vi "TestiLabview2LowLevel.vi"() -> ()   [LabVIEW 2018]
uses:
  <vilib>/vision/Image Controls.llb/IMAQ Image.ctl
  <vilib>/vision/driver/Vision Acquisition Express Utility VIs.llb/Vision Acquisition Path Convert (Path).vi
  <vilib>/vision/NI_Vision_Development_Module.lvlib
panel:
  out "Isbjerg spottet":i32[](array[numeric])
  out "Y":dbl[][](array[numeric])
  out "X":dbl[][](array[numeric])
  out "Image":T1(plugin-control)
  out "Array":cluster{"X Centroid":sgl, "Y Centroid":sgl}[](array[cluster])
  # "Tager isbjerge i rækkefølgen: y: 0 -> 480"
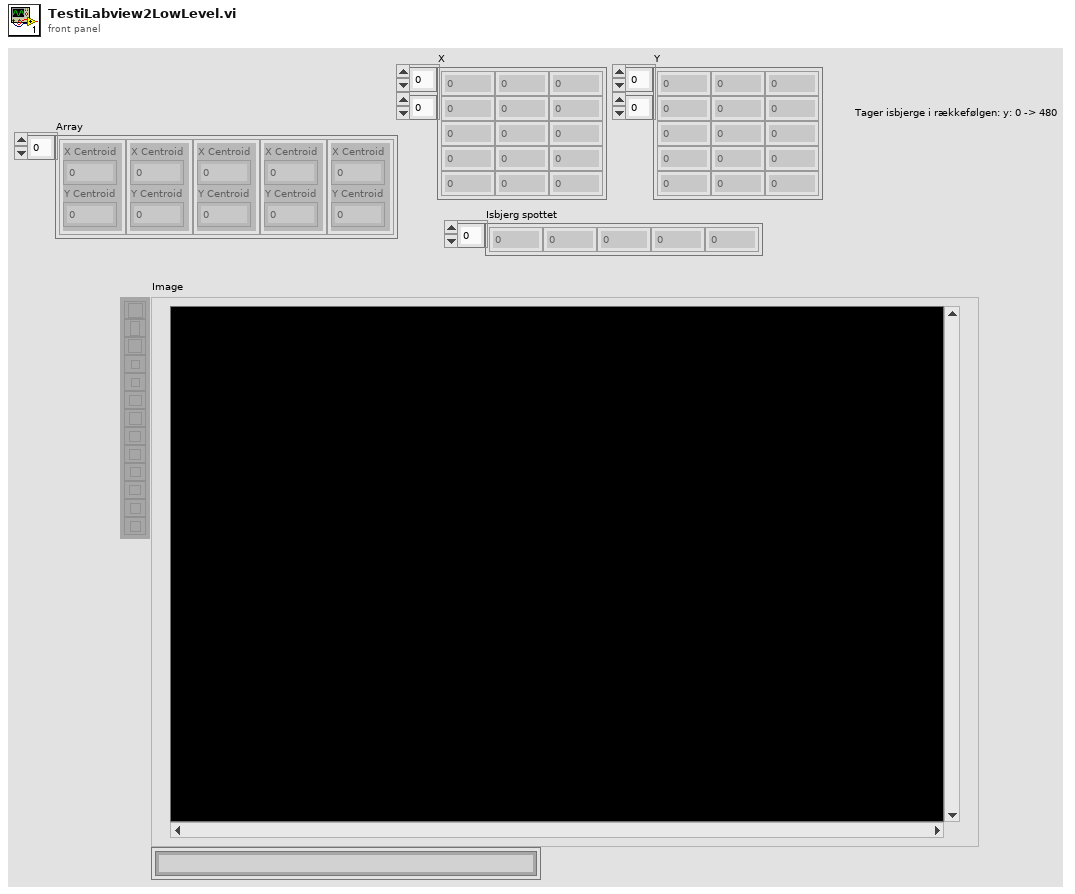
[diagram p1: front panel]
types:
  T1 = typedef "IMAQ Image.ctl" = refnum<image>
  T2 = typedef "Image Type" = u32
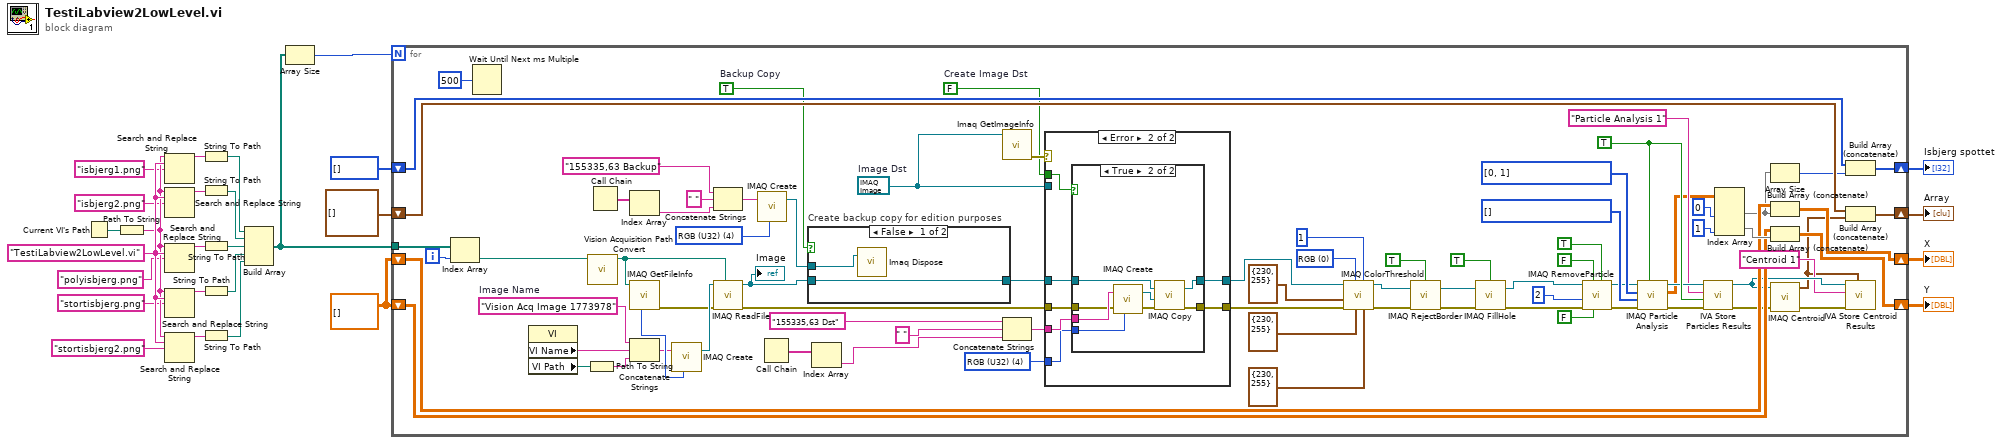
[diagram p0: block diagram]
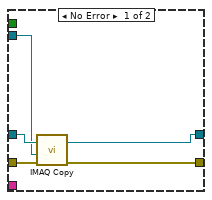
[diagram p2: hidden frame]
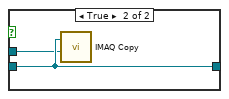
[diagram p4: hidden frame]
diagram:
  w10 = "TestiLabview2LowLevel.vi" ("search string")
  w25 = dbl[][] []
  n1 = Current VI's Path() -> (path=w19:path)
  n2 = Path To String(path=w19) -> (string=w9:string)
  n3 = Search and Replace String(input string=w9, search string=w10, replace string="isbjerg1.png" ("search string")) -> (result string=w18:string)  [unwired: 5 in, 3 out]
  n4 = Search and Replace String(input string=w9, search string=w10, replace string="isbjerg2.png" ("search string")) -> (result string=w17:string)  [unwired: 5 in, 3 out]
  n5 = Search and Replace String(input string=w9, search string=w10, replace string="polyisbjerg.png" ("search string")) -> (result string=w16:string)  [unwired: 5 in, 3 out]
  n6 = Search and Replace String(input string=w9, search string=w10, replace string="stortisbjerg.png" ("search string")) -> (result string=w15:string)  [unwired: 5 in, 3 out]
  n7 = Search and Replace String(input string=w9, search string=w10, replace string="stortisbjerg2.png" ("search string")) -> (result string=w14:string)  [unwired: 5 in, 3 out]
  n8 = String To Path(string=w18) -> (path=w11:path)
  n9 = String To Path(string=w17) -> (path=w12:path)
  n10 = String To Path(string=w16) -> (path=w2:path)
  n11 = String To Path(string=w15) -> (path=w13:path)
  n12 = String To Path(string=w14) -> (path=w1:path)
  n13 = Build Array(w11, w12, w2, w13, w1) -> (w3:path[])
  n14 = Array Size(array=w3) -> (size(s)=w21:i32)
  n15 = for {
    N: w21 -> [_]
    shift-right: [w106] -> w27
    shift-left: cluster{"X Centroid":sgl, "Y Centroid":sgl}[] [] -> [w105]
    tunnel: w3 -> [w103]
    shift-right: [w98] -> w24
    shift-left: w25 -> [w96]
    shift-right: [w97] -> w23
    shift-left: w25 -> [w95]
    shift-right: [w92] -> w20
    shift-left: i32[] [] -> [w91]
    i -> [w104]
    w79 = T1 refnum  # Image Dst
    w41 = i32[] [] items=["Center of Mass X", "Center of Mass Y", "First Pixel X", "First Pixel Y", "Bounding Rect Left", "Bounding Rect Top", "Bounding Rect Right", "Bounding Rect Bottom", "Max Feret Diameter Start X", "Max Feret Diameter Start Y", "Max Feret Diameter End X", "Max Feret Diameter End Y", "Max Horiz. Segment Length Left", "Max Horiz. Segment Length Right", "Max Horiz. Segment Length Row", "-", "Bounding Rect Width", "Bounding Rect Height", "Bounding Rect Diagonal", "Perimeter", "Convex Hull Perimeter", "Holes' Perimeter", "Max Feret Diameter", "Equivalent Ellipse Major Axis", "Equivalent Ellipse Minor Axis", "Equivalent Ellipse Minor Axis (Feret)", "Equivalent Rect Long Side", "Equivalent Rect Short Side", "Equivalent Rect Diagonal", "Equivalent Rect Short Side (Feret)", "Average Horiz. Segment Length", "Average Vert. Segment Length", "Hydraulic Radius", "Waddel Disk Diameter", "-", "Area", "Holes' Area", "Particle & Holes' Area", "Convex Hull Area", "Image Area", "-", "Number of Holes", "Number of Horiz. Segments", "Number of Vert. Segments", "-", "Orientation", "Max Feret Diameter Orientation", "-", "% Area/Image Area", "% Area/(Particle & Holes' Area)", "Ratio of Equivalent Ellipse Axes", "Ratio of Equivalent Rect Sides", "-", "Elongation Factor", "Compactness Factor", "Heywood Circularity Factor", "Type Factor", "-", "Sum X", "Sum Y", "Sum XX", "Sum XY", "Sum YY", "Sum XXX", "Sum XXY", "Sum XYY", "Sum YYY", "-", "Moment of Inertia XX", "Moment of Inertia XY", "Moment of Inertia YY", "Moment of Inertia XXX", "Moment of Inertia XXY", "Moment of Inertia XYY", "Moment of Inertia YYY", "Norm. Moment of Inertia XX", "Norm. Moment of Inertia XY", "Norm. Moment of Inertia YY", "Norm. Moment of Inertia XXX", "Norm. Moment of Inertia XXY", "Norm. Moment of Inertia XYY", "Norm. Moment of Inertia YYY", "Hu Moment 1", "Hu Moment 2", "Hu Moment 3", "Hu Moment 4", "Hu Moment 5", "Hu Moment 6", "Hu Moment 7"] ("Real-World Measurements")
    w42 = i32[] [0, 1] items=["Center of Mass X", "Center of Mass Y", "First Pixel X", "First Pixel Y", "Bounding Rect Left", "Bounding Rect Top", "Bounding Rect Right", "Bounding Rect Bottom", "Max Feret Diameter Start X", "Max Feret Diameter Start Y", "Max Feret Diameter End X", "Max Feret Diameter End Y", "Max Horiz. Segment Length Left", "Max Horiz. Segment Length Right", "Max Horiz. Segment Length Row", "-", "Bounding Rect Width", "Bounding Rect Height", "Bounding Rect Diagonal", "Perimeter", "Convex Hull Perimeter", "Holes' Perimeter", "Max Feret Diameter", "Equivalent Ellipse Major Axis", "Equivalent Ellipse Minor Axis", "Equivalent Ellipse Minor Axis (Feret)", "Equivalent Rect Long Side", "Equivalent Rect Short Side", "Equivalent Rect Diagonal", "Equivalent Rect Short Side (Feret)", "Average Horiz. Segment Length", "Average Vert. Segment Length", "Hydraulic Radius", "Waddel Disk Diameter", "-", "Area", "Holes' Area", "Particle & Holes' Area", "Convex Hull Area", "Image Area", "-", "Number of Holes", "Number of Horiz. Segments", "Number of Vert. Segments", "-", "Orientation", "Max Feret Diameter Orientation", "-", "% Area/Image Area", "% Area/(Particle & Holes' Area)", "Ratio of Equivalent Ellipse Axes", "Ratio of Equivalent Rect Sides", "-", "Elongation Factor", "Compactness Factor", "Heywood Circularity Factor", "Type Factor", "-", "Sum X", "Sum Y", "Sum XX", "Sum XY", "Sum YY", "Sum XXX", "Sum XXY", "Sum XYY", "Sum YYY", "-", "Moment of Inertia XX", "Moment of Inertia XY", "Moment of Inertia YY", "Moment of Inertia XXX", "Moment of Inertia XXY", "Moment of Inertia XYY", "Moment of Inertia YYY", "Norm. Moment of Inertia XX", "Norm. Moment of Inertia XY", "Norm. Moment of Inertia YY", "Norm. Moment of Inertia XXX", "Norm. Moment of Inertia XXY", "Norm. Moment of Inertia XYY", "Norm. Moment of Inertia YYY", "Hu Moment 1", "Hu Moment 2", "Hu Moment 3", "Hu Moment 4", "Hu Moment 5", "Hu Moment 6", "Hu Moment 7"] ("Pixel Measurements")
    w39 = TRUE ("Connectivity 4/8 (8)")
    w60 = u16 0 items=["RGB", "HSL", "HSV", "HSI"] ("Color Mode")
    w62 = T2 4 items=["Grayscale (U8)", "Grayscale (I16)", "Grayscale (SGL)", "Complex (CSG)", "RGB (U32)", "HSL (U32)", "RGB (U64)", "Grayscale (U16)"] ("Image Dst Type")
    w63 = T2 4 items=["Grayscale (U8)", "Grayscale (I16)", "Grayscale (SGL)", "Complex (CSG)", "RGB (U32)", "HSL (U32)", "RGB (U64)", "Grayscale (U16)"] ("Image Type")
    w80 = TRUE  # Backup Copy
    w75 = FALSE  # Create Image Dst
    w84 = "Vision Acq Image 1773978"  # Image Name
    n16 = Index Array(array=w103, index=w104) -> (element=w81:path)
    n17 = Wait Until Next ms Multiple(millisecond multiple=u32 500) -> ()  [unwired: 1 out]
    n18 = property class="VI"() -> ("VI Name"=w86:string, "VI Path"=w87:path)  [unwired: 2 in, 2 out]
    n19 = Path To String(path=w87) -> (string=w85:string)
    n20 = call-poly <vilib>:"Vision Acquisition Path Convert.vi"("Path In"=w81) -> ("Path Out"=w82:path)  [unwired: 10 in]
    n21 = Call Chain() -> (call chain=w69:string[])
    n22 = Index Array(array=w69) -> (element=w68:string)  [unwired: 1 in]
    n23 = call "IMAQ GetFileInfo"("File Path"=w82) -> ("error out"=w88:errorcluster, "Image Type"=w89:T2)  [unwired: 1 in, 8 out]
    n24 = Concatenate Strings(w84, w86, w85) -> (w83:string)
    n25 = call "IMAQ Create"("Image Name"=w83, "Image Type"=w89) -> ("New Image"=w90:T1)  [unwired: 2 in, 2 out]
    n26 = Concatenate Strings("155335,63 Backup" ("Backup Image Name"), " ", w68) -> (w65:string)
    n27 = call "IMAQ ReadFile"("File Path"=w82, "error in (no error)"=w88, "Image"=w90) -> ("error out"=w30:errorcluster, "Image Out"=w31:T1)  [unwired: 2 in, 5 out]
    "Image" <- w31
    n28 = call "IMAQ Create"("Image Name"=w65, "Image Type"=w63) -> ("New Image"=w64:T1)  [unwired: 2 in, 2 out]
    n29 = Call Chain() -> (call chain=w74:string[])
    n30 = case "Create backup copy for edition purposes" shown="False" w80 {
      tunnel: [w130 w132] -> w77
      tunnel: w31 -> [w130 w132]
      tunnel: w64 -> [w129 w131]
      frame False {
        n31 = call "Imaq Dispose"("Image"=w129) -> ()  [unwired: 2 in, 4 out]
      }
      frame True {
        n32 = call "IMAQ Copy"("Image Dst"=w131, "Image Src"=w132) -> ()  [unwired: 1 in, 5 out]
      }
    }
    n33 = Index Array(array=w74) -> (element=w72:string)  [unwired: 1 in]
    n34 = call "Imaq GetImageInfo"("Image"=w79) -> ("error out"=w78:errorcluster)  [unwired: 1 in, 9 out]
    n35 = Concatenate Strings("155335,63 Dst" ("Image Dst Name"), " ", w72) -> (w70:string)
    n36 = case shown="Error" w78 {
      tunnel: [w111 w115] -> w56
      tunnel: [w110 w114] -> w76
      tunnel: w77 -> [w109 w116]
      tunnel: w30 -> [w108 w112]
      tunnel: w79 -> [w107 _]
      tunnel: w70 -> [_ w118]
      tunnel: w62 -> [_ w117]
      tunnel: w75 -> [_ w113]
      frame No Error {
        n37 = call "IMAQ Copy"("error in (no error)"=w108, "Image Dst"=w107, "Image Src"=w109) -> ("error out"=w110:errorcluster, "Image Dst Out"=w111:T1)  [unwired: 3 out]
      }
      frame Error {
        n38 = case shown="True" w113 {
          tunnel: w118 -> [_ w128]
          tunnel: w117 -> [_ w127]
          tunnel: w116 -> [w120 w125]
          tunnel: [w120 w124] -> w115
          tunnel: [w119 w123] -> w114
          tunnel: w112 -> [w119 w121]
          frame False {
          }
          frame True {
            n39 = call "IMAQ Create"("Image Name"=w128, "Image Type"=w127, "error in (no error)"=w121) -> ("New Image"=w126:T1, "error out"=w122:errorcluster)  [unwired: 1 in, 1 out]
            n40 = call "IMAQ Copy"("error in (no error)"=w122, "Image Dst"=w126, "Image Src"=w125) -> ("error out"=w123:errorcluster, "Image Dst Out"=w124:T1)  [unwired: 3 out]
          }
        }
      }
    }
    n41 = call "IMAQ ColorThreshold"("Blue or Luma or Val or Inten Range"=cluster{"Lower value":i32, "Upper value":i32} {"Lower value"=230, "Upper value"=255}, "Replace Value"=1, "Green or Sat Range"=cluster{"Lower value":i32, "Upper value":i32} {"Lower value"=230, "Upper value"=255}, "Color Mode"=w60, "error in (no error)"=w76, "Red or Hue Range"=cluster{"Lower value":i32, "Upper value":i32} {"Lower value"=230, "Upper value"=255}, "Image Src"=w56) -> ("error out"=w55:errorcluster, "Image Dst Out"=w53:T1)  [unwired: 1 in, 2 out]
    n42 = call "IMAQ RejectBorder"("error in (no error)"=w55, "Image Src"=w53, "Connectivity 4/8 (8)"=TRUE) -> ("error out"=w52:errorcluster, "Image Dst Out"=w50:T1)  [unwired: 1 in, 2 out]
    n43 = call "IMAQ FillHole"("error in (no error)"=w52, "Image Src"=w50, "Connectivity 4/8 (8)"=TRUE) -> ("error out"=w49:errorcluster, "Image Dst Out"=w44:T1)  [unwired: 1 in, 2 out]
    n44 = call "IMAQ RemoveParticle"("Connectivity 4/8 (8)"=TRUE, "Low Pass/High Pass (Low)"=FALSE, "Square/Hexa (Square)"=FALSE, "error in (no error)"=w49, "Number of Erosion"=2, "Image Src"=w44) -> ("error out"=w43:errorcluster, "Image Dst Out"=w40:T1)  [unwired: 1 in, 3 out]
    n45 = call "IMAQ Particle Analysis"("Connectivity 4/8 (8)"=w39, "error in (no error)"=w43, "Real-World Measurements"=w41, "Pixel Measurements"=w42, "Image"=w40) -> ("error out"=w36:errorcluster, "Particle Measurements (Pixels)"=w29:dbl[][], "Image Out (duplicate)"=w38:T1)  [unwired: 4 out]
    n46 = call <vilib>:"IVA Store Particles Results.vi"("error in (no error)"=w36, "Connectivity 4/8 (8)"=w39, "Step Name"="Particle Analysis 1", "Image in"=w38) -> ("error out"=w35:errorcluster, "Image dup"=w33:T1)  [unwired: 6 out]
    n47 = Index Array(array=w29, index (col) #1=0 ("index (col)"), index (col) #2=1 ("index (col)")) -> (element #1=w94:dbl[], element #2=w99:dbl[])  [unwired: 2 in]
    n48 = Array Size(array=w94) -> (size(s)=w93:i32)
    n49 = Build Array (concatenate)(w96, w94) -> (w98:dbl[][])
    n50 = Build Array (concatenate)(w95, w99) -> (w97:dbl[][])
    n51 = call "IMAQ Centroid"("error in (no error)"=w35, "Image"=w33) -> ("error out"=w34:errorcluster, "Centroid"=w28:cluster{"X Centroid":sgl, "Y Centroid":sgl})  [unwired: 1 in, 1 out]
    n52 = Build Array (concatenate)(w91, w93) -> (w92:i32[])
    n53 = Build Array (concatenate)(w105, w28) -> (w106:cluster{"X Centroid":sgl, "Y Centroid":sgl}[])
    n54 = call <vilib>:"IVA Store Centroid Results.vi"("Centroid in"=w28, "error in (no error)"=w34, "Step Name"="Centroid 1", "Image in"=w33) -> ()  [unwired: 8 out]
  }
  "Array" <- w27
  "X" <- w24
  "Y" <- w23
  "Isbjerg spottet" <- w20
